vi "Datasheet S#P Channel Data.vi"(1 "Channel Data":T1[](array[typedef])) -> (0 "HTM Table Rows":string)   [LabVIEW 2011]
uses:
  TDMS/TDMS Channel (Sxx).ctl
  www/tests/S Parameter/TypeDefs/SP Format.ctl
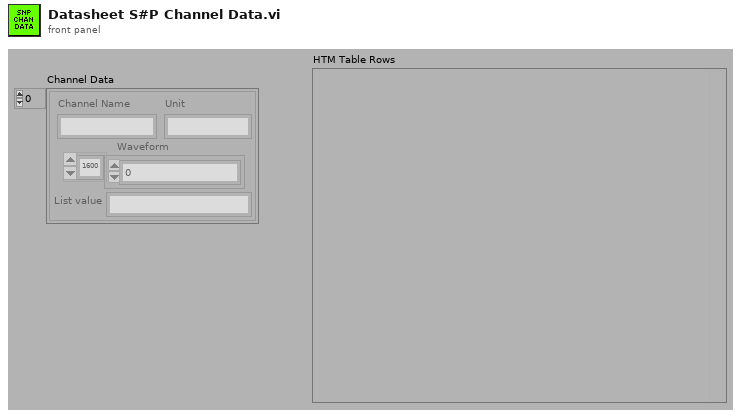
[diagram p1: front panel]
types:
  T1 = typedef "TDMS Channel (Sxx).ctl" = cluster{"Channel Name":string, "Waveform":dbl[], "Unit":string, "List value":string}
  T2 = typedef "SP Format.ctl" = enum16{"Log Mag", "Lin Mag", "SWR", "Phase", "Expanded Phase", "Delay", "Insertion Loss", "Isolation", "Return Loss"}
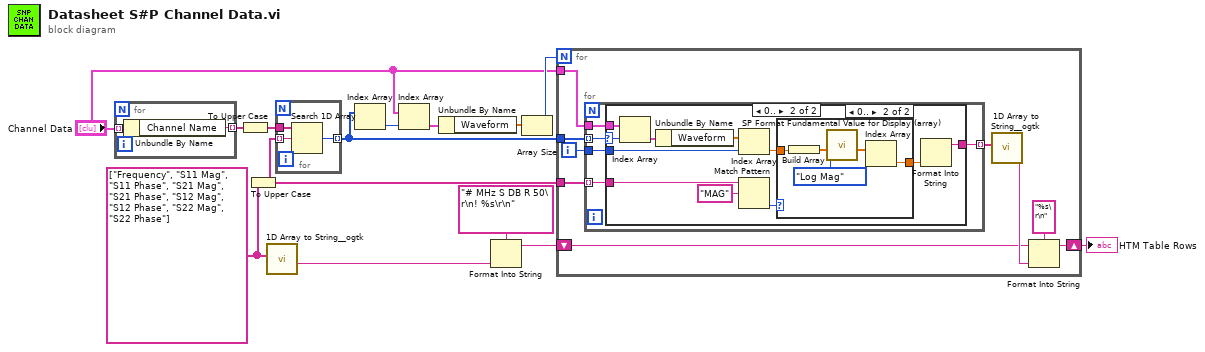
[diagram p0: block diagram]
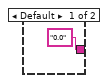
[diagram p2: hidden frame]
diagram:
  w5 = string[] ["Frequency", "S11 Mag", "S11 Phase", "S21 Mag", "S21 Phase", "S12 Mag", "S12 Phase", "S22 Mag", "S22 Phase"]
  n1 = for {
    tunnel: "Channel Data" -> [w16] mode=indexing
    tunnel: [w15] -> w13 mode=indexing
    n2 = Unbundle By Name(w16) -> ("Channel Name"=w15:string)
  }
  n3 = To Upper Case(1:w13) -> (0:w12:string[])
  n4 = To Upper Case(1:w5) -> (0:w4:string[])
  n5 = call "1D Array to String__ogtk.vi"("Array of Strings"=w5) -> ("delimited string"=w1:string)  [unwired: 10 in]
  n6 = for {
    tunnel: w12 -> [w19]
    tunnel: w4 -> [w18] mode=indexing
    tunnel: [w17] -> w11 mode=indexing
    n7 = Search 1D Array(1D array=w19, element=w18) -> (index of element=w17:i32)  [unwired: 1 in]
  }
  n8 = Index Array(array=w11) -> (element=w10:i32)  [unwired: 1 in]
  n9 = Index Array(array="Channel Data", index=w10) -> (element=w9:T1)
  n10 = Unbundle By Name(w9) -> ("Waveform"=w8:dbl[])
  n11 = Format Into String(format string="# MHz S DB R 50\r\n! %s\r\n", w1) -> (resulting string=w2:string)  [unwired: 2 in, 1 out]
  n12 = Array Size(array=w8) -> (size(s)=w7:i32)
  n13 = for {
    N: w7 -> [_]
    tunnel: w11 -> [w28]
    shift-right: [w21] -> w14
    shift-left: w2 -> [w22]
    tunnel: "Channel Data" -> [w27]
    tunnel: w4 -> [w20]
    i -> [w26]
    n14 = for {
      tunnel: w28 -> [w33] mode=indexing
      tunnel: w27 -> [w32]
      tunnel: w26 -> [w31]
      tunnel: [w30] -> w25 mode=indexing
      tunnel: w20 -> [w29] mode=indexing
      n15 = case shown="0.." w33 {
        selector: w33 -> [_ w43]
        tunnel: w32 -> [_ w44]
        tunnel: w31 -> [_ w41]
        tunnel: ["0.0" w40] -> w30
        tunnel: w29 -> [_ w39]
        frame Default {
        }
        frame 0.. {
          n16 = Index Array(array=w44, index=w43) -> (element=w45:T1)
          n17 = Unbundle By Name(w45) -> ("Waveform"=w42:dbl[])
          n18 = Index Array(array=w42, index=w41) -> (element=w36:dbl)
          n19 = Match Pattern(string=w39, regular expression="MAG") -> (offset past match=w37:i32)  [unwired: 1 in, 3 out]
          n20 = case shown="0.." w37 {
            tunnel: w36 -> [w46 w51]
            tunnel: [w46 w48] -> w35
            frame Default {
            }
            frame 0.. {
              n21 = Build Array(w51) -> (w49:dbl[])
              n22 = call "SP Format Fundamental Value for Display (array).vi"("Display Format"=SP_Format."Log Mag", "Fundamental Values"=w49) -> ("Formatted Values"=w50:dbl[])  [unwired: 9 in]
              n23 = Index Array(array=w50) -> (element=w48:dbl)  [unwired: 1 in]
            }
          }
          n24 = Format Into String(w35) -> (resulting string=w40:string)  [unwired: 3 in, 1 out]
        }
      }
    }
    n25 = call "1D Array to String__ogtk.vi"("Array of Strings"=w25) -> ("delimited string"=w23:string)  [unwired: 10 in]
    n26 = Format Into String(format string="%s\r\n", initial string=w22, w23) -> (resulting string=w21:string)  [unwired: 1 in, 1 out]
  }
  "HTM Table Rows" <- w14
